vi "Query Keys.vi"(8 "error in (no error)":errorcluster, 9 "timeout_ms":u64=2000, 10 "Query Expression":string, 11 "Zenoh in":refnum<class "Zenoh.lvclass">) -> (0 "error out":errorcluster, 3 "Query Key Return":T1 {"Data Bytes" format="%.0x"; "Key Bytes" format="%.0x"})   [LabVIEW 2021, in "Zenoh.lvclass"]
uses:
  Zenoh.lvclass
  typedef/Query Keys Return.ctl
  Zenoh.lvclass/Zenoh.ctl
  SubVIs/Add Zenoh Error.vi
  <vilib>/CIF Foundation/CIF Utilities/Errors/Append Error Location.vi
  SubVIs/Get Zenoh Path.vi
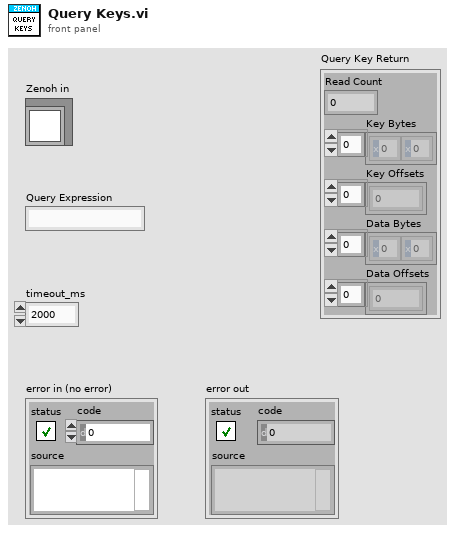
[diagram p1: front panel]
types:
  T1 = typedef "Zenoh.lvclass/Query Keys Return.ctl" = cluster{"Read Count":i32, "Key Bytes":u8[], "Key Offsets":u32[], "Data Bytes":u8[], "Data Offsets":u32[]}
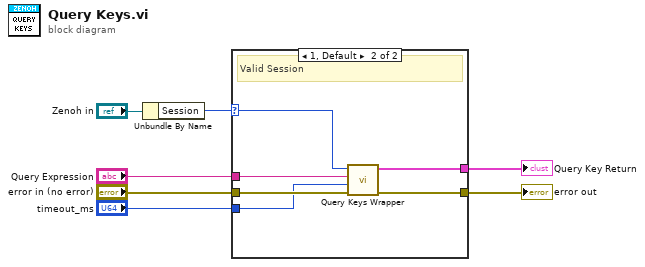
[diagram p0: block diagram]
diagram:
  n1 = Unbundle By Name("Zenoh in") -> ("Session"=w5:u64)
  n2 = case shown="1, Default" w5 {
    selector: w5 -> [_ w12]
    tunnel: "Query Expression" -> [_ w11]
    tunnel: "error in (no error)" -> [w8 w14]
    tunnel: [w8 w13] -> w4
    tunnel: "timeout_ms" -> [_ w10]
    tunnel: [_ w9] -> w1
    frame 0 {
      # "Invalid session"
    }
    frame 1, Default {
      # "Valid Session"
      n3 = call "Query Keys Wrapper.vi"("error in (no error)"=w14, "timeout_ms"=w10, "key_expr"=w11, "Reader Handle"=w12) -> ("error out"=w13:errorcluster, "Query Key Return"=w9:T1)  [unwired: 6 in]
    }
  }
  "error out" <- w4
  "Query Key Return" <- w1
